vi "RemoteControlFifoImage.vi"() -> ()   [LabVIEW 2023]
doc: "This VI demonstrates how a Becker&Hickl compiled application can be remotely controlled by using the LabVIEW VI-Server.\nFifoImage.exe has opened a port at 3366. The functional global variable ControlFifoImage.vi is obtaining and keeping references to selected front panel controls in FifoImage.exe and allows read and write functionality on those.\nRemote controlling can be done from the LabVIEW development environment or a compiled application. With slight modifications controlling can be done over a network.\n\ninfo@becker-hickl.com"
uses:
  Example_Controls/UserInput.ctl
panel:
  out "FifoImage Result message":string
  in  "Init":bool
  out "2D Picture":picture
  in  "Stop":bool
  in  "CenterOfMass":bool
  in  "SaveMeas":bool
  in  "StopMeas":bool
  in  "StartMeas":bool
  in  "ClearImage":bool
  in  "UserInput":T1={"tac_range"=50.0, "tac_gain"=1, "tac_offset"=0.0, "tac_limit_high"=10.0, "tac_limit_low"=80.0, "collect_time"=0.01, "sync_threshold"=-20.0, "sync_zc_level"=0.0, "sync_freq_div"=1, "cfd_limit_low"=0.0, "cfd_zc_level"=0.0} {"sync_freq_div" items=["1"=1, "2"=2, "4"=4]; "cfd_zc_level" min=-96 max=96 step=0.1 format="%#_3g"; "cfd_limit_low" min=-500 max=0 step=0.1 format="%#_3g"; "sync_zc_level" min=-96 max=96 step=0.1 format="%#_3g"; "sync_threshold" min=-500 max=-20 step=0.1 format="%#_3g"; "tac_limit_low" format="%.3g"; "tac_limit_high" min=0 max=100 step=0.1 format="%.3g"; "collect_time" min=1e-07 max=100000 step=0.001; "tac_offset" min=0 max=100 step=0.1 format="%.4g"; "tac_gain" min=1 max=15 step=1; "tac_range" format="%^#_6g"}
  # "This VI demonstrates how a Becker&Hickl compiled application can be remotely\ncontrolled by using the LabVIEW VI-Server.\nFifoImage.exe has opened a port at 3366. The functional global variable \nControlFifoImage.vi is obtaining and keeping references to selected front panel\ncontrols in FifoImage.exe and allows read and write functionality on those.\nRemote controlling can be done from the LabVIEW development environment or\na compiled application. With slight modifications controlling can be done over \na network."
  # "TAC / Time Range"
  # "CFD"
  # "(start)"
  # "SYNC"
  # "(stop)"
  # "range"
  # "gain"
  # "threshold(LL)"
  # "offset"
  # "limit high"
  # "limit low"
  # "zero cross(ZC)"
  # "Collection Time"
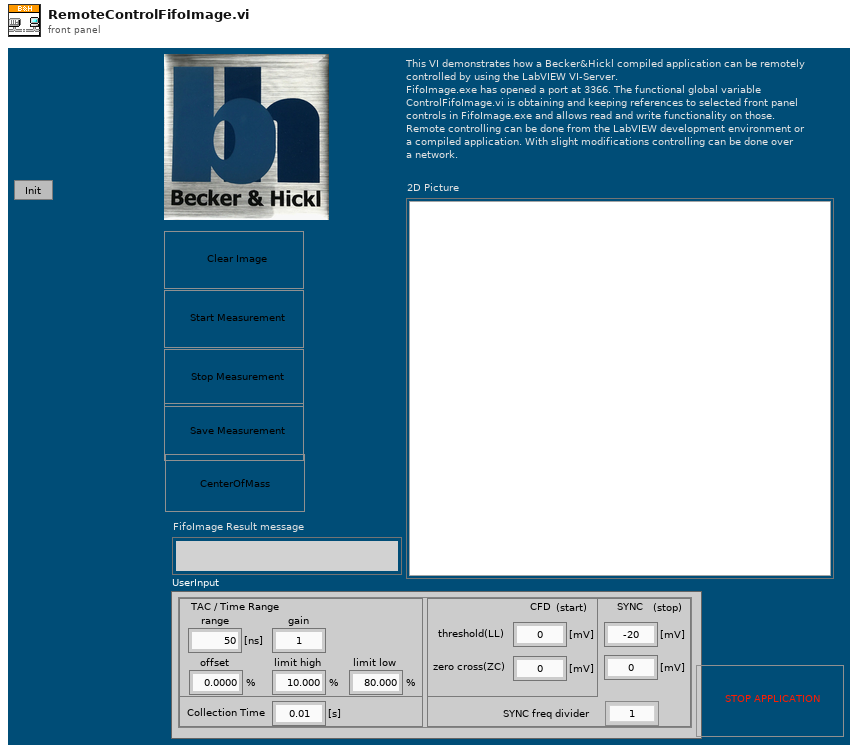
[diagram p1: front panel]
types:
  T1 = typedef "UserInput.ctl" = cluster{"tac_range":sgl, "tac_gain":i16, "tac_offset":sgl, "tac_limit_high":sgl, "tac_limit_low":sgl, "collect_time":sgl, "sync_threshold":sgl, "sync_zc_level":sgl, "sync_freq_div":i16, "cfd_limit_low":sgl, "cfd_zc_level":sgl}
  T2 = cluster{refnum<vi>, refnum<vi>, refnum<vi>, refnum<vi>, refnum<vi>}
  T3 = typedef "imagedata.ctl" = cluster{"image type":i32, "image depth":i32, "image":u8[], "mask":u8[], "colors":u32[], "Rectangle":cluster{"left":i16, "top":i16, "right":i16, "bottom":i16}}
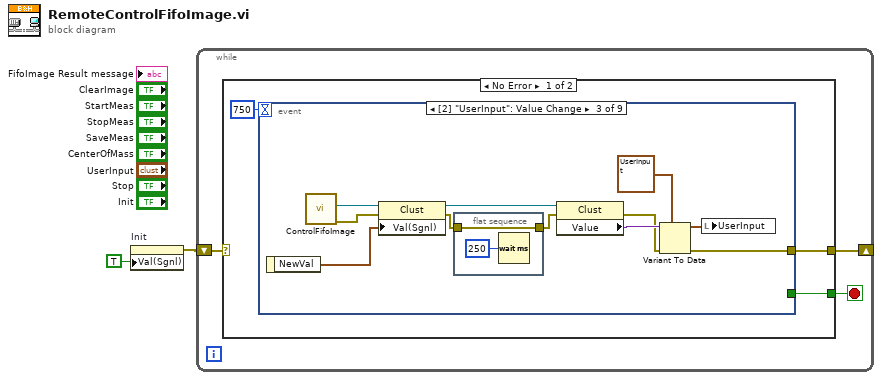
[diagram p0: block diagram]
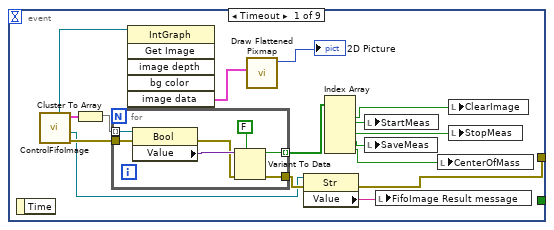
[diagram p2: hidden frame]
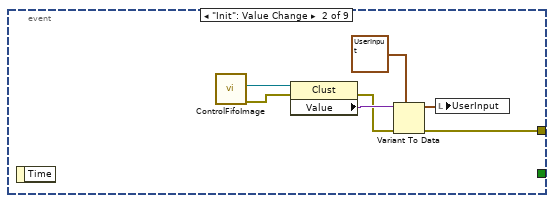
[diagram p3: hidden frame]
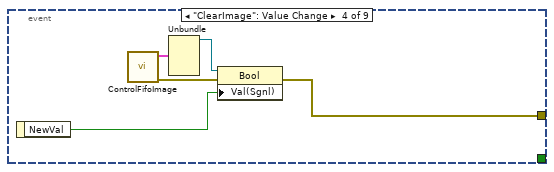
[diagram p4: hidden frame]
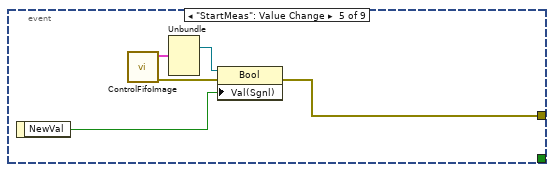
[diagram p5: hidden frame]
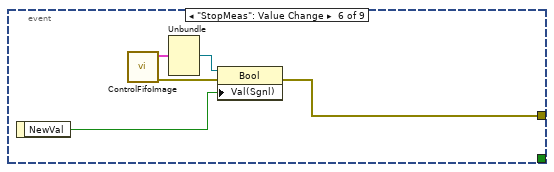
[diagram p6: hidden frame]
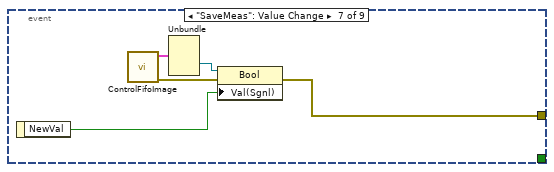
[diagram p7: hidden frame]
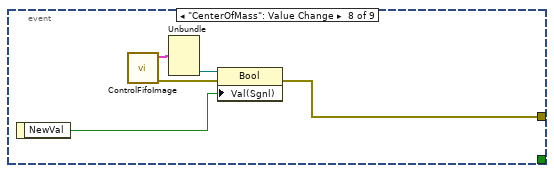
[diagram p8: hidden frame]
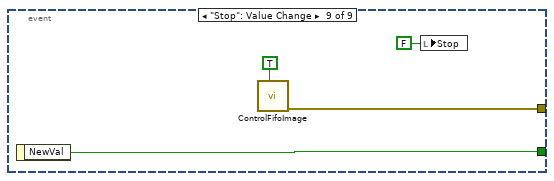
[diagram p9: hidden frame]
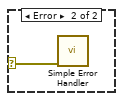
[diagram p10: hidden frame]
diagram:
  n1 = property on="Init" class="Bool (strict)"("Val(Sgnl)"=TRUE ("Value (Signaling)")) -> (error out=w2:errorcluster)  [unwired: 2 in, 1 out]
  n2 = while {
    shift-right: [w5] -> _
    shift-left: w2 -> [w4]
    stop <- w3 stop-if-true
    n3 = case shown="No Error" w4 {
      selector: w4 -> [_ w81]
      tunnel: [w8 _] -> w5
      tunnel: [w7 _] -> w3
      frame No Error {
        n4 = event shown="[2] \"UserInput\": Value Change" {
          selector: _ -> [_ _ _ _ _ _ _ _ _]
          dyn-events: _ -> [_ _ _ _ _ _ _ _ _]
          timeout: 750 -> [_ _ _ _ _ _ _ _ _]
          tunnel: [w11 w34 w40 w52 w58 w63 w68 w73 w77] -> w8
          tunnel: [_ _ _ _ _ _ _ _ w80] -> w7
          event Timeout {
            n5 = event-data() -> ()  [unwired: 1 in, 1 out]
            n6 = call "ControlFifoImage.vi"() -> ("ErrorOut"=w21:errorcluster, "ResultCtlRef"=w9:refnum<vi>, "ButtonRefs"=w23:T2, "IntensityImageRef"=w15:refnum<vi>)  [unwired: 7 in, 1 out]
            n7 = Cluster To Array(cluster=w23) -> (array=w22:refnum<vi>[])
            n8 = for {
              tunnel: [w30] -> w24 mode=indexing
              tunnel: [w28] -> w10
              tunnel: w22 -> [w26] mode=indexing
              tunnel: w21 -> [w25]
              n9 = property class="Bool"(reference=w26, error in=w25) -> (error out=w29:errorcluster, "Value"=w31:variant)  [unwired: 1 out]
              n10 = Variant To Data(error in=w29, type=FALSE, Variant=w31) -> (data=w30:bool, error out=w28:errorcluster)
            }
            n11 = invoke class="IntGraph" method="Get Image"(reference=w15) -> ("image data"=w14:T3)  [unwired: 5 in, 5 out]
            n12 = call <vilib>:"Draw Flattened Pixmap.vi"("image data"=w14) -> ("new picture"=→"2D Picture":picture)  [unwired: 8 in]
            n13 = property class="Str"(reference=w9, error in=w10) -> (error out=w11:errorcluster, "Value"=w12:string)  [unwired: 1 out]
            n14 = Index Array(array=w24) -> (element #1=w20:bool, element #2=w19:bool, element #3=w18:bool, element #4=w17:bool, element #5=w16:bool)  [unwired: 5 in]
            n15 = local write "StartMeas"(w19) -> ()
            n16 = local write "SaveMeas"(w17) -> ()
            n17 = local write "FifoImage Result message"(w12) -> ()
            n18 = local write "CenterOfMass"(w16) -> ()
            n19 = local write "ClearImage"(w20) -> ()
            n20 = local write "StopMeas"(w18) -> ()
          }
          event "Init": Value Change {
            n21 = event-data() -> ()  [unwired: 1 in, 1 out]
            n22 = call "ControlFifoImage.vi"() -> ("ErrorOut"=w32:errorcluster, "UserInputRef"=w33:refnum<vi>)  [unwired: 7 in, 3 out]
            n23 = property class="Clust"(reference=w33, error in=w32) -> (error out=w35:errorcluster, "Value"=w38:variant)  [unwired: 1 out]
            n24 = Variant To Data(error in=w35, type=T1 {"tac_range"=50.0, "tac_gain"=1, "tac_offset"=0.0, "tac_limit_high"=10.0, "tac_limit_low"=80.0, "collect_time"=0.01, "sync_threshold"=-20.0, "sync_zc_level"=0.0, "sync_freq_div"=1, "cfd_limit_low"=0.0, "cfd_zc_level"=0.0} ("User Input"), Variant=w38) -> (data=w36:T1, error out=w34:errorcluster)
            n25 = local write "UserInput"(w36) -> ()
          }
          event Value Change {
            n26 = event-data() -> ("NewVal"=w39:T1)  [unwired: 1 in]
            n27 = call "ControlFifoImage.vi"() -> ("ErrorOut"=w44:errorcluster, "UserInputRef"=w47:refnum<vi>)  [unwired: 7 in, 3 out]
            n28 = property class="Clust"(reference=w47, error in=w44, "Val(Sgnl)"=w39) -> (reference out=w46:refnum<vi>, error out=w42:errorcluster)
            n29 = flat-sequence {
              tunnel: w42 -> [w50]
              tunnel: [w50] -> w41
              frame #0 {
                n30 = Wait (ms)(milliseconds to wait=u32 250) -> ()  [unwired: 1 out]
              }
            }
            n31 = property class="Clust"(reference=w46, error in=w41) -> (error out=w43:errorcluster, "Value"=w49:variant)  [unwired: 1 out]
            n32 = Variant To Data(error in=w43, type=T1 {"tac_range"=50.0, "tac_gain"=1, "tac_offset"=0.0, "tac_limit_high"=10.0, "tac_limit_low"=80.0, "collect_time"=0.01, "sync_threshold"=-20.0, "sync_zc_level"=0.0, "sync_freq_div"=1, "cfd_limit_low"=0.0, "cfd_zc_level"=0.0} ("User Input"), Variant=w49) -> (data=w45:T1, error out=w40:errorcluster)
            n33 = local write "UserInput"(w45) -> ()
          }
          event "ClearImage": Value Change {
            n34 = event-data() -> ("NewVal"=w55:bool)  [unwired: 1 in]
            n35 = call "ControlFifoImage.vi"() -> ("ErrorOut"=w56:errorcluster, "ButtonRefs"=w54:T2)  [unwired: 7 in, 3 out]
            n36 = Unbundle(w54) -> (w53:refnum<vi>)  [unwired: 4 out]
            n37 = property class="Bool"(reference=w53, error in=w56, "Val(Sgnl)"=w55) -> (error out=w52:errorcluster)  [unwired: 1 out]
          }
          event "StartMeas": Value Change {
            n38 = event-data() -> ("NewVal"=w60:bool)  [unwired: 1 in]
            n39 = call "ControlFifoImage.vi"() -> ("ErrorOut"=w61:errorcluster, "ButtonRefs"=w59:T2)  [unwired: 7 in, 3 out]
            n40 = Unbundle(w59) -> (w57:refnum<vi>)  [unwired: 4 out]
            n41 = property class="Bool"(reference=w57, error in=w61, "Val(Sgnl)"=w60) -> (error out=w58:errorcluster)  [unwired: 1 out]
          }
          event "StopMeas": Value Change {
            n42 = event-data() -> ("NewVal"=w65:bool)  [unwired: 1 in]
            n43 = call "ControlFifoImage.vi"() -> ("ErrorOut"=w66:errorcluster, "ButtonRefs"=w64:T2)  [unwired: 7 in, 3 out]
            n44 = Unbundle(w64) -> (w62:refnum<vi>)  [unwired: 4 out]
            n45 = property class="Bool"(reference=w62, error in=w66, "Val(Sgnl)"=w65) -> (error out=w63:errorcluster)  [unwired: 1 out]
          }
          event "SaveMeas": Value Change {
            n46 = event-data() -> ("NewVal"=w70:bool)  [unwired: 1 in]
            n47 = call "ControlFifoImage.vi"() -> ("ErrorOut"=w71:errorcluster, "ButtonRefs"=w69:T2)  [unwired: 7 in, 3 out]
            n48 = Unbundle(w69) -> (w67:refnum<vi>)  [unwired: 4 out]
            n49 = property class="Bool"(reference=w67, error in=w71, "Val(Sgnl)"=w70) -> (error out=w68:errorcluster)  [unwired: 1 out]
          }
          event "CenterOfMass": Value Change {
            n50 = event-data() -> ("NewVal"=w75:bool)  [unwired: 1 in]
            n51 = call "ControlFifoImage.vi"() -> ("ErrorOut"=w76:errorcluster, "ButtonRefs"=w74:T2)  [unwired: 7 in, 3 out]
            n52 = Unbundle(w74) -> (w72:refnum<vi>)  [unwired: 4 out]
            n53 = property class="Bool"(reference=w72, error in=w76, "Val(Sgnl)"=w75) -> (error out=w73:errorcluster)  [unwired: 1 out]
          }
          event "Stop": Value Change {
            n54 = event-data() -> ("NewVal"=w80:bool)  [unwired: 1 in]
            n55 = call "ControlFifoImage.vi"("CloseReferences(F)"=TRUE) -> ("ErrorOut"=w77:errorcluster)  [unwired: 6 in, 4 out]
            n56 = local write "Stop"(FALSE ("Stop")) -> ()
          }
        }
      }
      frame Error {
        n57 = call <vilib>:"Simple Error Handler.vi"("error in (no error)"=w81) -> ()  [unwired: 4 in, 5 out]
      }
    }
  }
